vi "Receive Messenger.vi"(8 "error in (no error)":errorcluster, 10 "Messenger In":refnum<class "Messenger.lvclass">, 11 "Root Actor in":refnum<class "Root Actor.lvclass">) -> (0 "error out":errorcluster, 3 "Root Actor out":refnum<class "Root Actor.lvclass">)   [LabVIEW 2024, in "Root Actor.lvclass"]
uses:
  Root Actor.lvclass
  C:/Users/iio/Desktop/Bussiness/Tricorn Re/Madelbrot 4.0/General Library/Ancestor Class/Actor/System Actor/System Actor.lvclass
  Messenger/Messenger/Messenger.lvclass
  Root Actor.lvclass/Root Actor.ctl
  System Actor/System Actor.lvclass/System Actor.ctl
  System Actor/Protected Data/Write Messenger Reference.vi
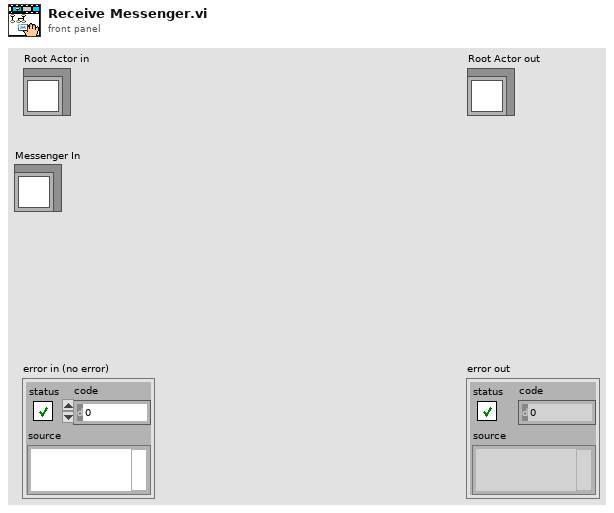
[diagram p1: front panel]
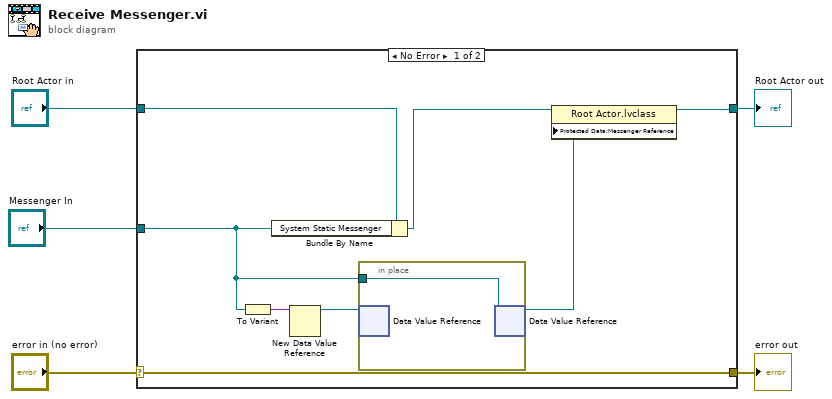
[diagram p0: block diagram]
diagram:
  n1 = case shown="No Error" "error in (no error)" {
    selector: "error in (no error)" -> [w13 w16]
    tunnel: [w13 w16] -> w4
    tunnel: [w10 w15] -> w2
    tunnel: "Root Actor in" -> [w12 w15]
    tunnel: "Messenger In" -> [w6 _]
    frame No Error {
      n2 = To Variant(anything=w6) -> (Variant=w9:variant)
      n3 = Bundle By Name(cluster=w12, "System Static Messenger"=w6) -> (w11:refnum<class "Root Actor.lvclass">)
      n4 = New Data Value Reference(data value=w9) -> (data value reference=w8:refnum<data-value>)  [unwired: 1 in, 1 out]
      n5 = in-place {
        in-place-border: w6 -> [w14]
        n6 = in-place-dvr #1(w8) -> ()  [unwired: 2 out]
        n7 = in-place-dvr #1(w14) -> (w7:refnum<data-value>)  [unwired: 1 out]
      }
      n8 = property class="Root Actor.lvclass"(reference=w11, "Protected Data:Messenger Reference"=w7) -> (reference out=w10:refnum<class "Root Actor.lvclass">)  [unwired: 1 in, 1 out]
    }
    frame Error {
    }
  }
  "error out" <- w4
  "Root Actor out" <- w2
